vi "SMTP Mail.vi"(8 "error in (no error)":errorcluster, 10 "Data":T1, 11 "Configure Server":T2={"Outgoing Mail Server (SMTP)"="smtp.gmail.com", "Port"="587", "Sender's Email Address"="ltt24012025@gmail.com", "username"="ltt24012025@gmail.com", "password"="hhib mwaf mimz fohz", "Enable TLS"=TRUE}) -> (0 "error out":errorcluster)   [LabVIEW 2023, in "HardwareAbstractionLayer_LVOOP.lvlib" / "Mail.lvclass"]
uses:
  Mail.lvclass
  Mail.lvclass/Mail.ctl
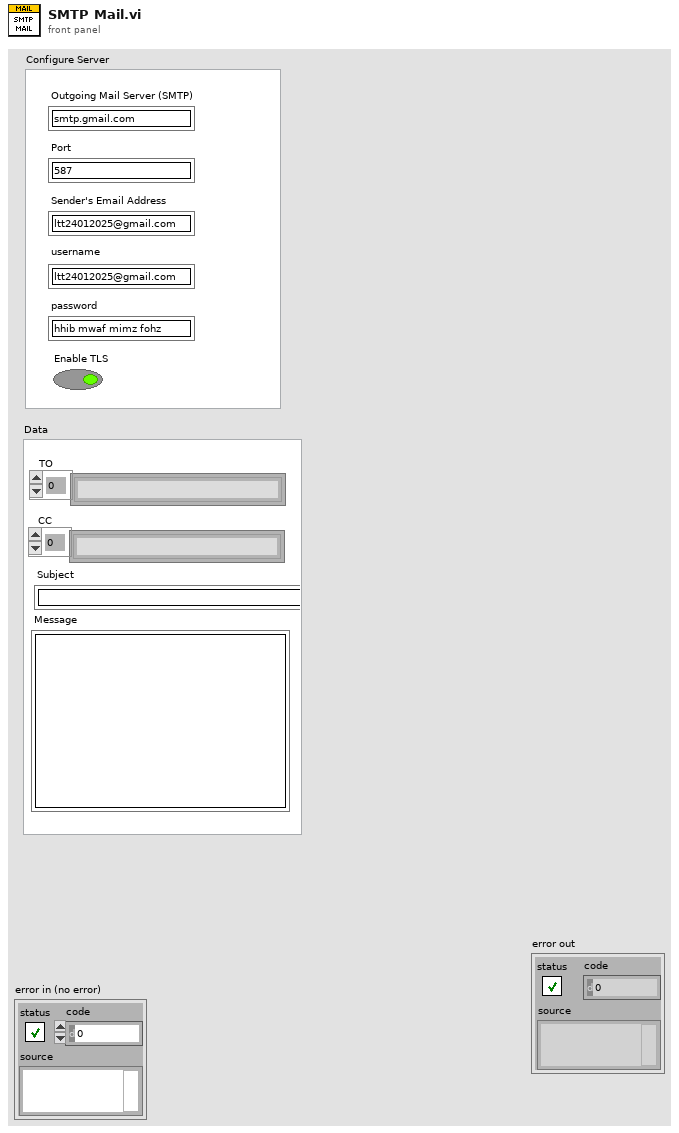
[diagram p1: front panel]
types:
  T1 = cluster{"TO":string[], "CC":string[], "Subject":string, "Message":string}
  T2 = cluster{"Outgoing Mail Server (SMTP)":string, "Port":string, "Sender's Email Address":string, "username":string, "password":string, "Enable TLS":bool}
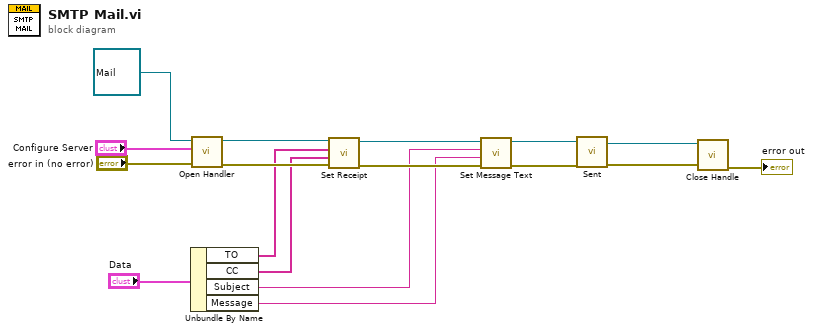
[diagram p0: block diagram]
diagram:
  n1 = Unbundle By Name("Data") -> ("TO"=w4:string[], "CC"=w3:string[], "Subject"=w2:string, "Message"=w1:string)
  n2 = call-dynamic "Open Handler.vi"("error in (no error)"="error in (no error)", "Configure Server"="Configure Server", "Mail in"=refnum<class "Mail.lvclass"> refnum) -> ("error out"=w15:errorcluster, "Mail out"=w16:refnum<class "Mail.lvclass">)  [unwired: 7 in]
  n3 = call-dynamic "Set Receipt.vi"("error in (no error)"=w15, "CC"=w3, "TO"=w4, "Mail in"=w16) -> ("error out"=w14:errorcluster, "Mail out"=w9:refnum<class "Mail.lvclass">)  [unwired: 6 in]
  n4 = call-dynamic "Set Message Text.vi"("error in (no error)"=w14, "Message"=w1, "Subject"=w2, "Mail in"=w9) -> ("error out"=w13:errorcluster, "Mail out"=w10:refnum<class "Mail.lvclass">)  [unwired: 6 in]
  n5 = call-dynamic "Sent.vi"("error in (no error)"=w13, "Mail in"=w10) -> ("error out"=w12:errorcluster, "Mail out"=w11:refnum<class "Mail.lvclass">)  [unwired: 8 in]
  n6 = call-dynamic "Close Handle.vi"("error in (no error)"=w12, "Mail in"=w11) -> ("error out"=→"error out":errorcluster)  [unwired: 8 in, 1 out]
